vi "2-4040_Set SampleNumber&AcquireData - Debug.vi"(8 "error in (no error)":errorcluster, 10 "Sample Number":i32, 11 "VISA resource name":refnum<visa-resource-name>) -> (0 "error out":errorcluster, 1 "Pressure":dbl[](array[numeric]), 2 "Tem":dbl[](array[numeric]), 3 "Flow":dbl[](array[numeric]), 5 "Time":string[](array[string]))   [LabVIEW 2017]
uses:
  <vilib>/Instr/_visa.llb/VISA Flush IO Buffer Mask.ctl
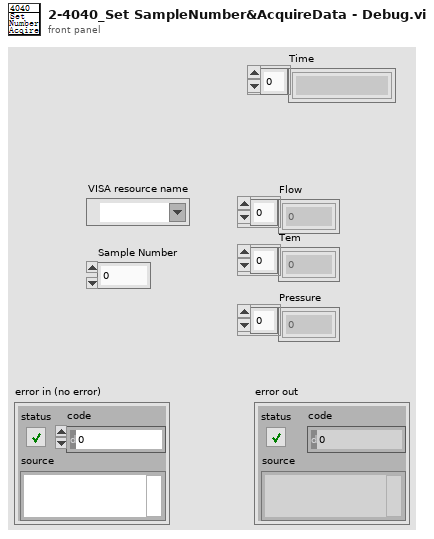
[diagram p1: front panel]
types:
  T1 = typedef "VISA Flush IO Buffer Mask.ctl" = u16
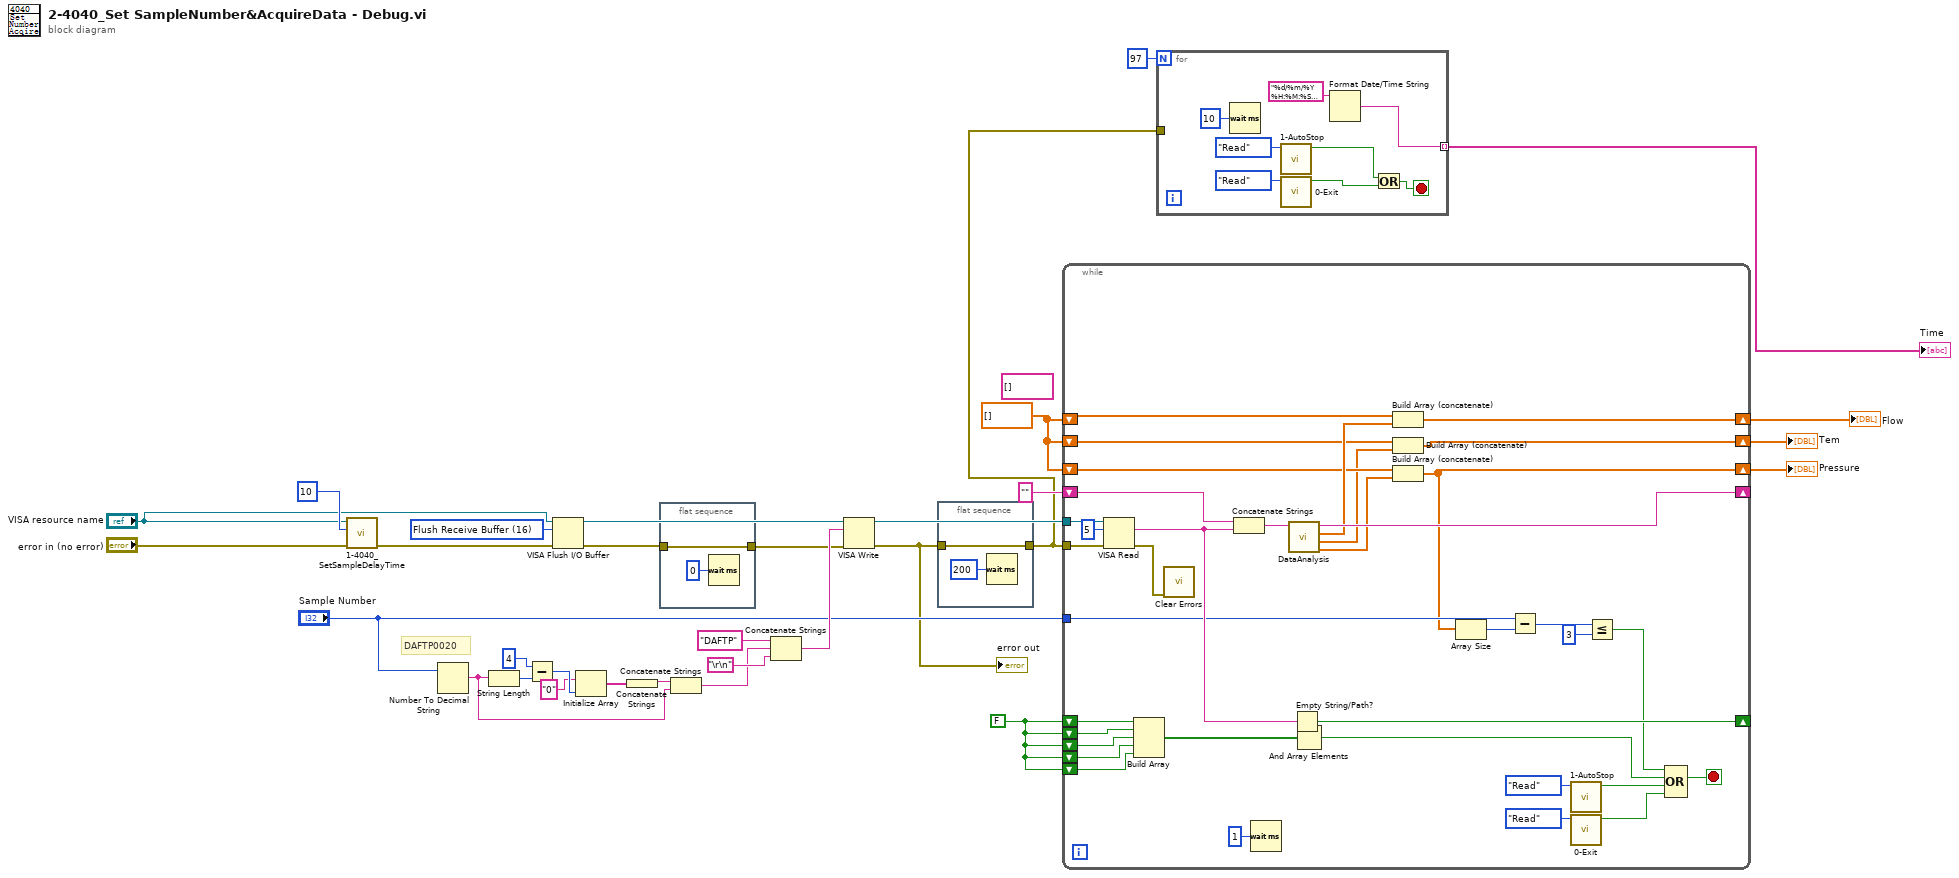
[diagram p0: block diagram]
diagram:
  (unwired) string[] []
  w12 = T1 16 items=["Flush Receive Buffer"=16, "Write Transmit Buffer to Device"=32, "Flush Receive Buffer (No I/O)"=64, "Flush Transmit Buffer"=128] ("Mask")
  w16 = dbl[] []
  w18 = FALSE
  # "DAFTP0020"
  n1 = call "1-4040_SetSampleDelayTime.vi"("Error in"="error in (no error)", "Sample Delay Time(ms)"=10 ("Delay Time"), "Visa IO"="VISA resource name") -> ("error out"=w5:errorcluster)  [unwired: 7 in, 1 out]
  n2 = Number To Decimal String(number="Sample Number") -> (decimal integer string=w23:string)  [unwired: 1 in]
  n3 = String Length(string=w23) -> (length=w29:i32)
  n4 = Subtract(x=4, y=w29) -> (x-y=w27:i32)
  n5 = VISA Flush I/O Buffer ("VISA清空I/O缓冲区")(VISA resource name="VISA resource name", mask (16)=w12, error in (no error)=w5) -> (VISA resource name out=w13:refnum<visa-resource-name>, error out=w11:errorcluster)
  n6 = Initialize Array("0", w27) -> (w25:string[])
  n7 = Concatenate Strings(w25) -> (w24:string)
  n8 = flat-sequence {
    tunnel: w11 -> [w33]
    tunnel: [w33] -> w10
    frame #0 {
      n9 = Wait (ms)(milliseconds to wait=u32 0) -> ()  [unwired: 1 out]
    }
  }
  n10 = Concatenate Strings(w24, w23) -> (w22:string)
  n11 = Concatenate Strings("DAFTP" ("写入缓冲区"), w22, "\r\n") -> (w21:string)
  n12 = VISA Write(VISA resource name=w13, write buffer=w21, error in (no error)=w10) -> (VISA resource name out=w20:refnum<visa-resource-name>, error out=w9:errorcluster)  [unwired: 1 out]
  "error out" <- w9
  n13 = flat-sequence {
    tunnel: w9 -> [w35]
    tunnel: [w35] -> w2
    frame #0 {
      n14 = Wait (ms)(milliseconds to wait=u32 200) -> ()  [unwired: 1 out]
    }
  }
  n15 = while {
    tunnel: w2 -> [w70]
    tunnel: w20 -> [w71]
    shift-right: [w66] -> _
    shift-left: "" -> [w68]
    shift-right: [w63] -> _
    shift-left: w18 -> [w62]
    shift-left: w18 -> [w61]
    shift-left: w18 -> [w60]
    shift-left: w18 -> [w59]
    shift-left: w18 -> [w58]
    tunnel: "Sample Number" -> [w53]
    shift-right: [w36] -> w4
    shift-left: w16 -> [w50]
    shift-right: [w38] -> w15
    shift-left: w16 -> [w48]
    shift-right: [w37] -> w14
    shift-left: w16 -> [w47]
    stop <- w52 stop-if-true
    n16 = VISA Read(VISA resource name=w71, byte count=u32 5 ("字节总数"), error in (no error)=w70) -> (read buffer=w64:string, error out=w65:errorcluster)  [unwired: 2 out]
    n17 = Build Array(w62, w61, w60, w59, w58) -> (w57:bool[])
    n18 = call <vilib>:"Clear Errors.vi"("error in (no error)"=w65) -> ()  [unwired: 5 in, 2 out]
    n19 = Concatenate Strings(w68, w64) -> (w67:string)
    n20 = Wait (ms)(milliseconds to wait=u32 1) -> ()  [unwired: 1 out]
    n21 = call "DataAnalysis.vi"("Data"=w67) -> ("3"=w45:dbl[], "2"=w46:dbl[], "1"=w49:dbl[], "Residue Datas"=w66:string)  [unwired: 6 in, 1 out]
    n22 = Empty String/Path?(string/path=w64) -> (empty?=w63:bool)
    n23 = And Array Elements(Boolean array=w57) -> (logical AND=w56:bool)
    n24 = Build Array (concatenate)(w50, w49) -> (w36:dbl[])
    n25 = Build Array (concatenate)(w48, w46) -> (w38:dbl[])
    n26 = Build Array (concatenate)(w47, w45) -> (w37:dbl[])
    n27 = Array Size(array=w37) -> (size(s)=w44:i32)
    n28 = Subtract(x=w53, y=w44) -> (x-y=w55:i32)
    n29 = call "1-AutoStop.vi"("Step"=enum16{"Initial", "Write", "Read"}."Read") -> ("AutoStop Out"=w40:bool)  [unwired: 9 in, 1 out]
    n30 = call "0-Exit.vi"("Step"=enum16{"Initial", "Write", "Read"}."Read") -> ("Exit Out"=w39:bool)  [unwired: 9 in, 1 out]
    n31 = Less Or Equal?(x=w55, y=3) -> (x <= y?=w51:bool)
    n32 = Compound Arithmetic op=OR(w51, w56, w40, w39) -> (w52:bool)
  }
  "Flow" <- w4
  "Tem" <- w15
  "Pressure" <- w14
  n33 = for {
    N: 97 -> [_]
    tunnel: w2 -> [_]
    tunnel: [w78] -> w1 mode=indexing
    stop <- w75 stop-if-true
    n34 = Wait (ms)(milliseconds to wait=u32 10 ("等待时间（毫秒）")) -> ()  [unwired: 1 out]
    n35 = call "1-AutoStop.vi"("Step"=enum16{"Initial", "Write", "Read"}."Read") -> ("AutoStop Out"=w74:bool)  [unwired: 9 in, 1 out]
    n36 = call "0-Exit.vi"("Step"=enum16{"Initial", "Write", "Read"}."Read") -> ("Exit Out"=w73:bool)  [unwired: 9 in, 1 out]
    n37 = Format Date/Time String(time format string (%c)="%d/%m/%Y %H:%M:%S%3u") -> (date/time string=w78:string)  [unwired: 2 in]
    n38 = Or(x=w74, y=w73) -> (x .or. y?=w75:bool)
  }
  "Time" <- w1
